vi "INVENTORY.vi"(9 "CURRENT_YEAR_DATA":string, 10 "ECODE 2":string, 11 "connection reference":T1) -> ()   [LabVIEW 2015]
uses:
  <vilib>/addons/database/Connection.llb/Conn ObjectReference.ctl
  <vilib>/Utility/miscctls.llb/LVRowAndColumnUnsignedTypeDef.ctl
  Controls/INVENTORY.ctl
  <vilib>/addons/database/Connection.llb/Conn Execute.vi
  <vilib>/addons/database/Recordset.llb/Rec Destroy - Connection.vi
  <vilib>/addons/database/_DB Variant To Data/Database Variant To Data.xnode
  <vilib>/addons/database/NI_Database_API.lvlib
  <vilib>/addons/database/Connection.llb/DB Tools Open Connec (String).vi
panel:
  out "COUNTER":dbl
  out "ECODE":string
  in  "QR_CODE (F2)":string
  in  "BOTTON_IMPORT":bool
  in  "BUTTON_EXIT":bool
  in  "Tab Control":enum32{"FROM CHECK STOCK", "FROM EXCEL FILE"}(tab)
  in  "Product":string(combo)
  in  "Path":path
  in  "NO.":string(combo)
  out "Table":string[][](table)
  # "INVENTORY"
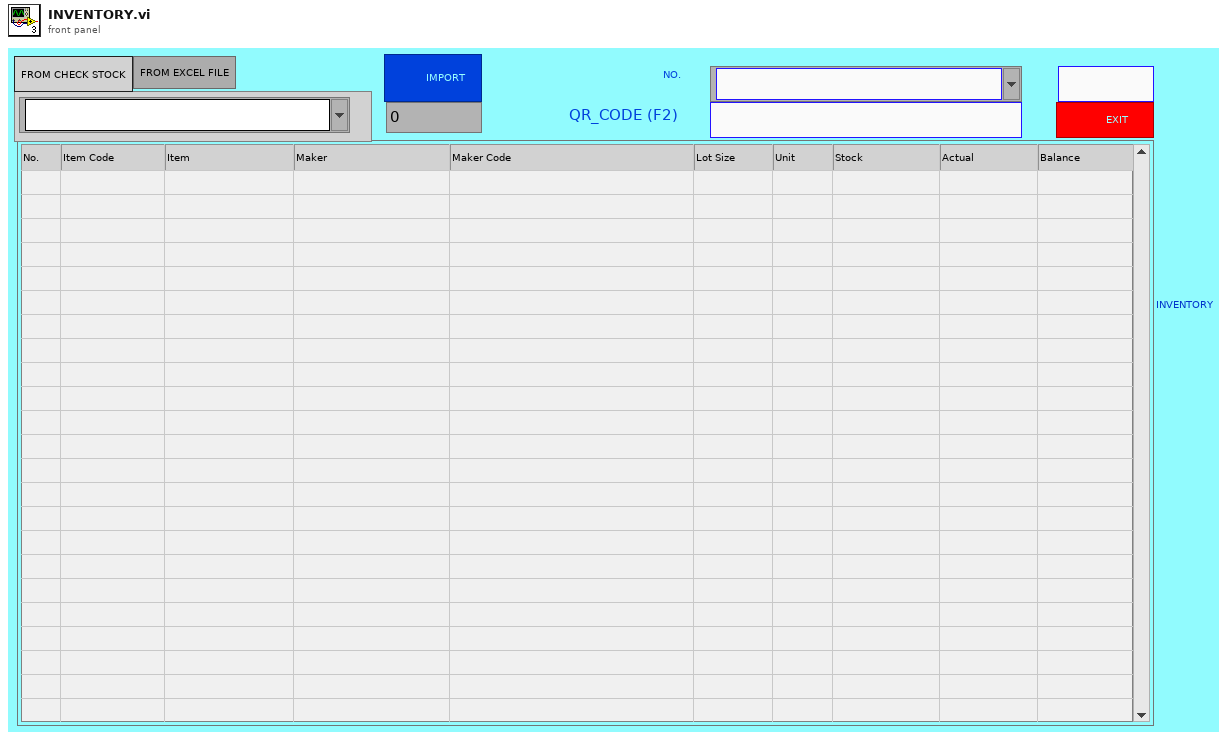
[diagram p1: front panel]
types:
  T1 = typedef "NI_Database_API.lvlib/Conn ObjectReference.ctl" = refnum<k1>
  T2 = typedef "LVRowAndColumnUnsignedTypeDef.ctl" = cluster{"Row":u32, "Column":u32}
  T3 = typedef "INVENTORY.ctl" = cluster{"ITEM_CODE":string, "PART_NAME":string, "MAKER":string, "PART_NO":string, "LOT_SIZE":dbl, "UNIT":string, "STOCK":dbl, "ACTUAL":dbl, "BALANCE":dbl}
  T4 = cluster{"QUANTITY":dbl, "INPUT_NO":string, "LINEBACK_NO":string, "OUTPUT_NO":string}[]
  T5 = cluster{"start (-1, -1)":cluster{"row":i32, "column":i32}, "end (-1, -1)":cluster{"row":i32, "column":i32}}
  T6 = cluster{"ITEM_CODE":string, "PART_NAME":string, "MAKER":string, "PART_NO":string, "LOT_SIZE":string, "UNIT":string, "STOCK":string, "ACTUAL":string, "BALANCE":string}
  T7 = cluster{"ITEM_CODE":string, "STOCK":dbl, "ACTUAL":dbl, "BALANCE":dbl}[]
  T8 = cluster{"seconds since 1Jan1904":timestamp, "NO.":string, "ECODE":string}
  T9 = typedef "NI_Database_API.lvlib/Rec ObjectReference.ctl" = refnum<k1>
  T10 = cluster{"seconds since 1Jan1904":timestamp, "String":string, "ECODE":string}
  T11 = cluster{"ITEM_CODE":string, "STOCK":dbl, "ACTUAL":dbl, "BALANCE":dbl}
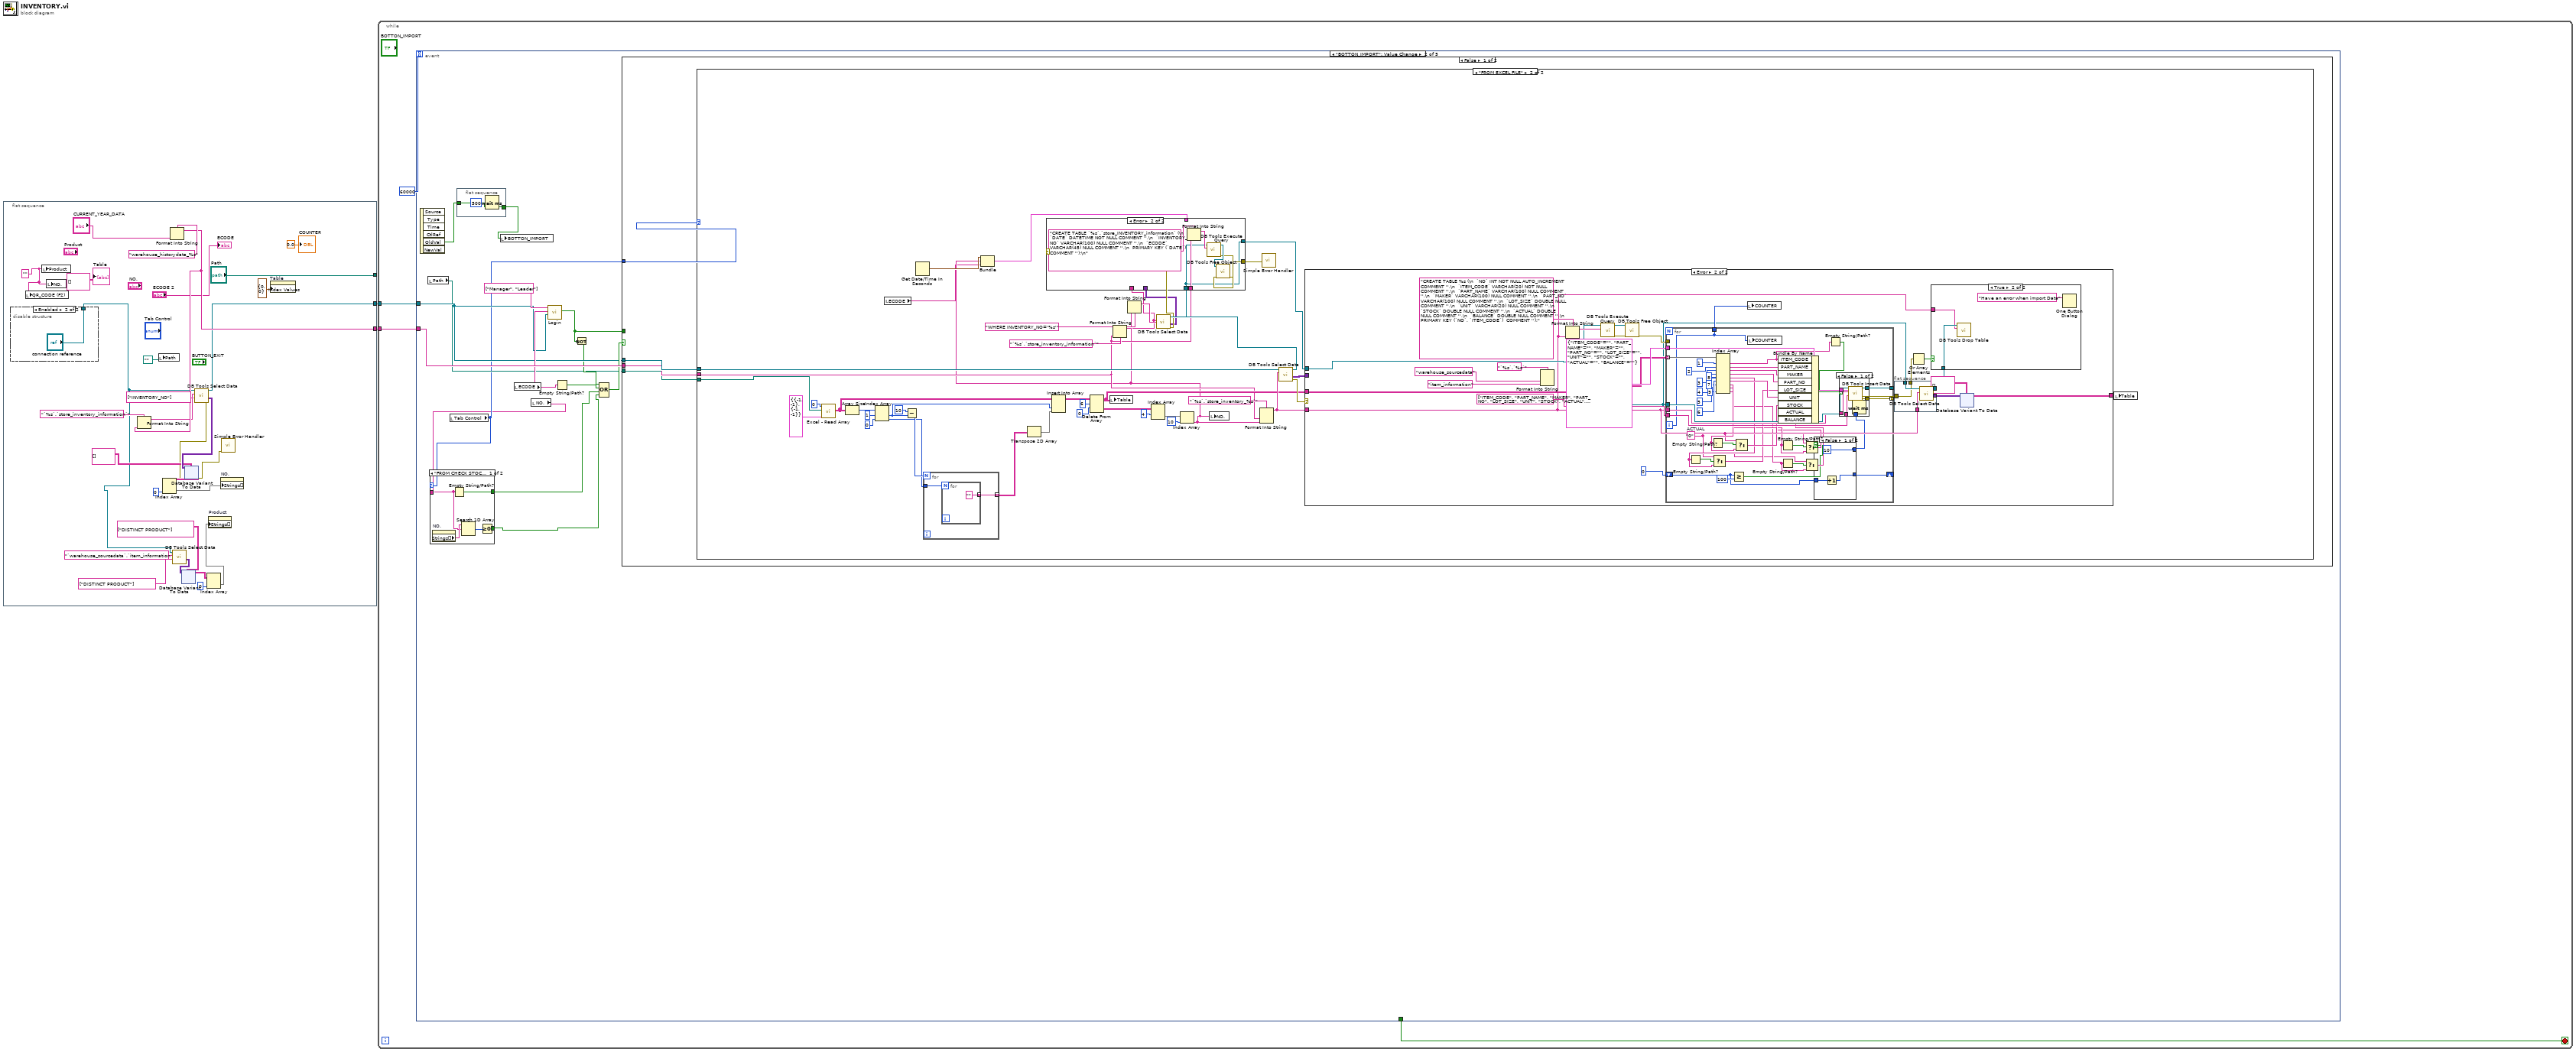
[diagram p0: block diagram]
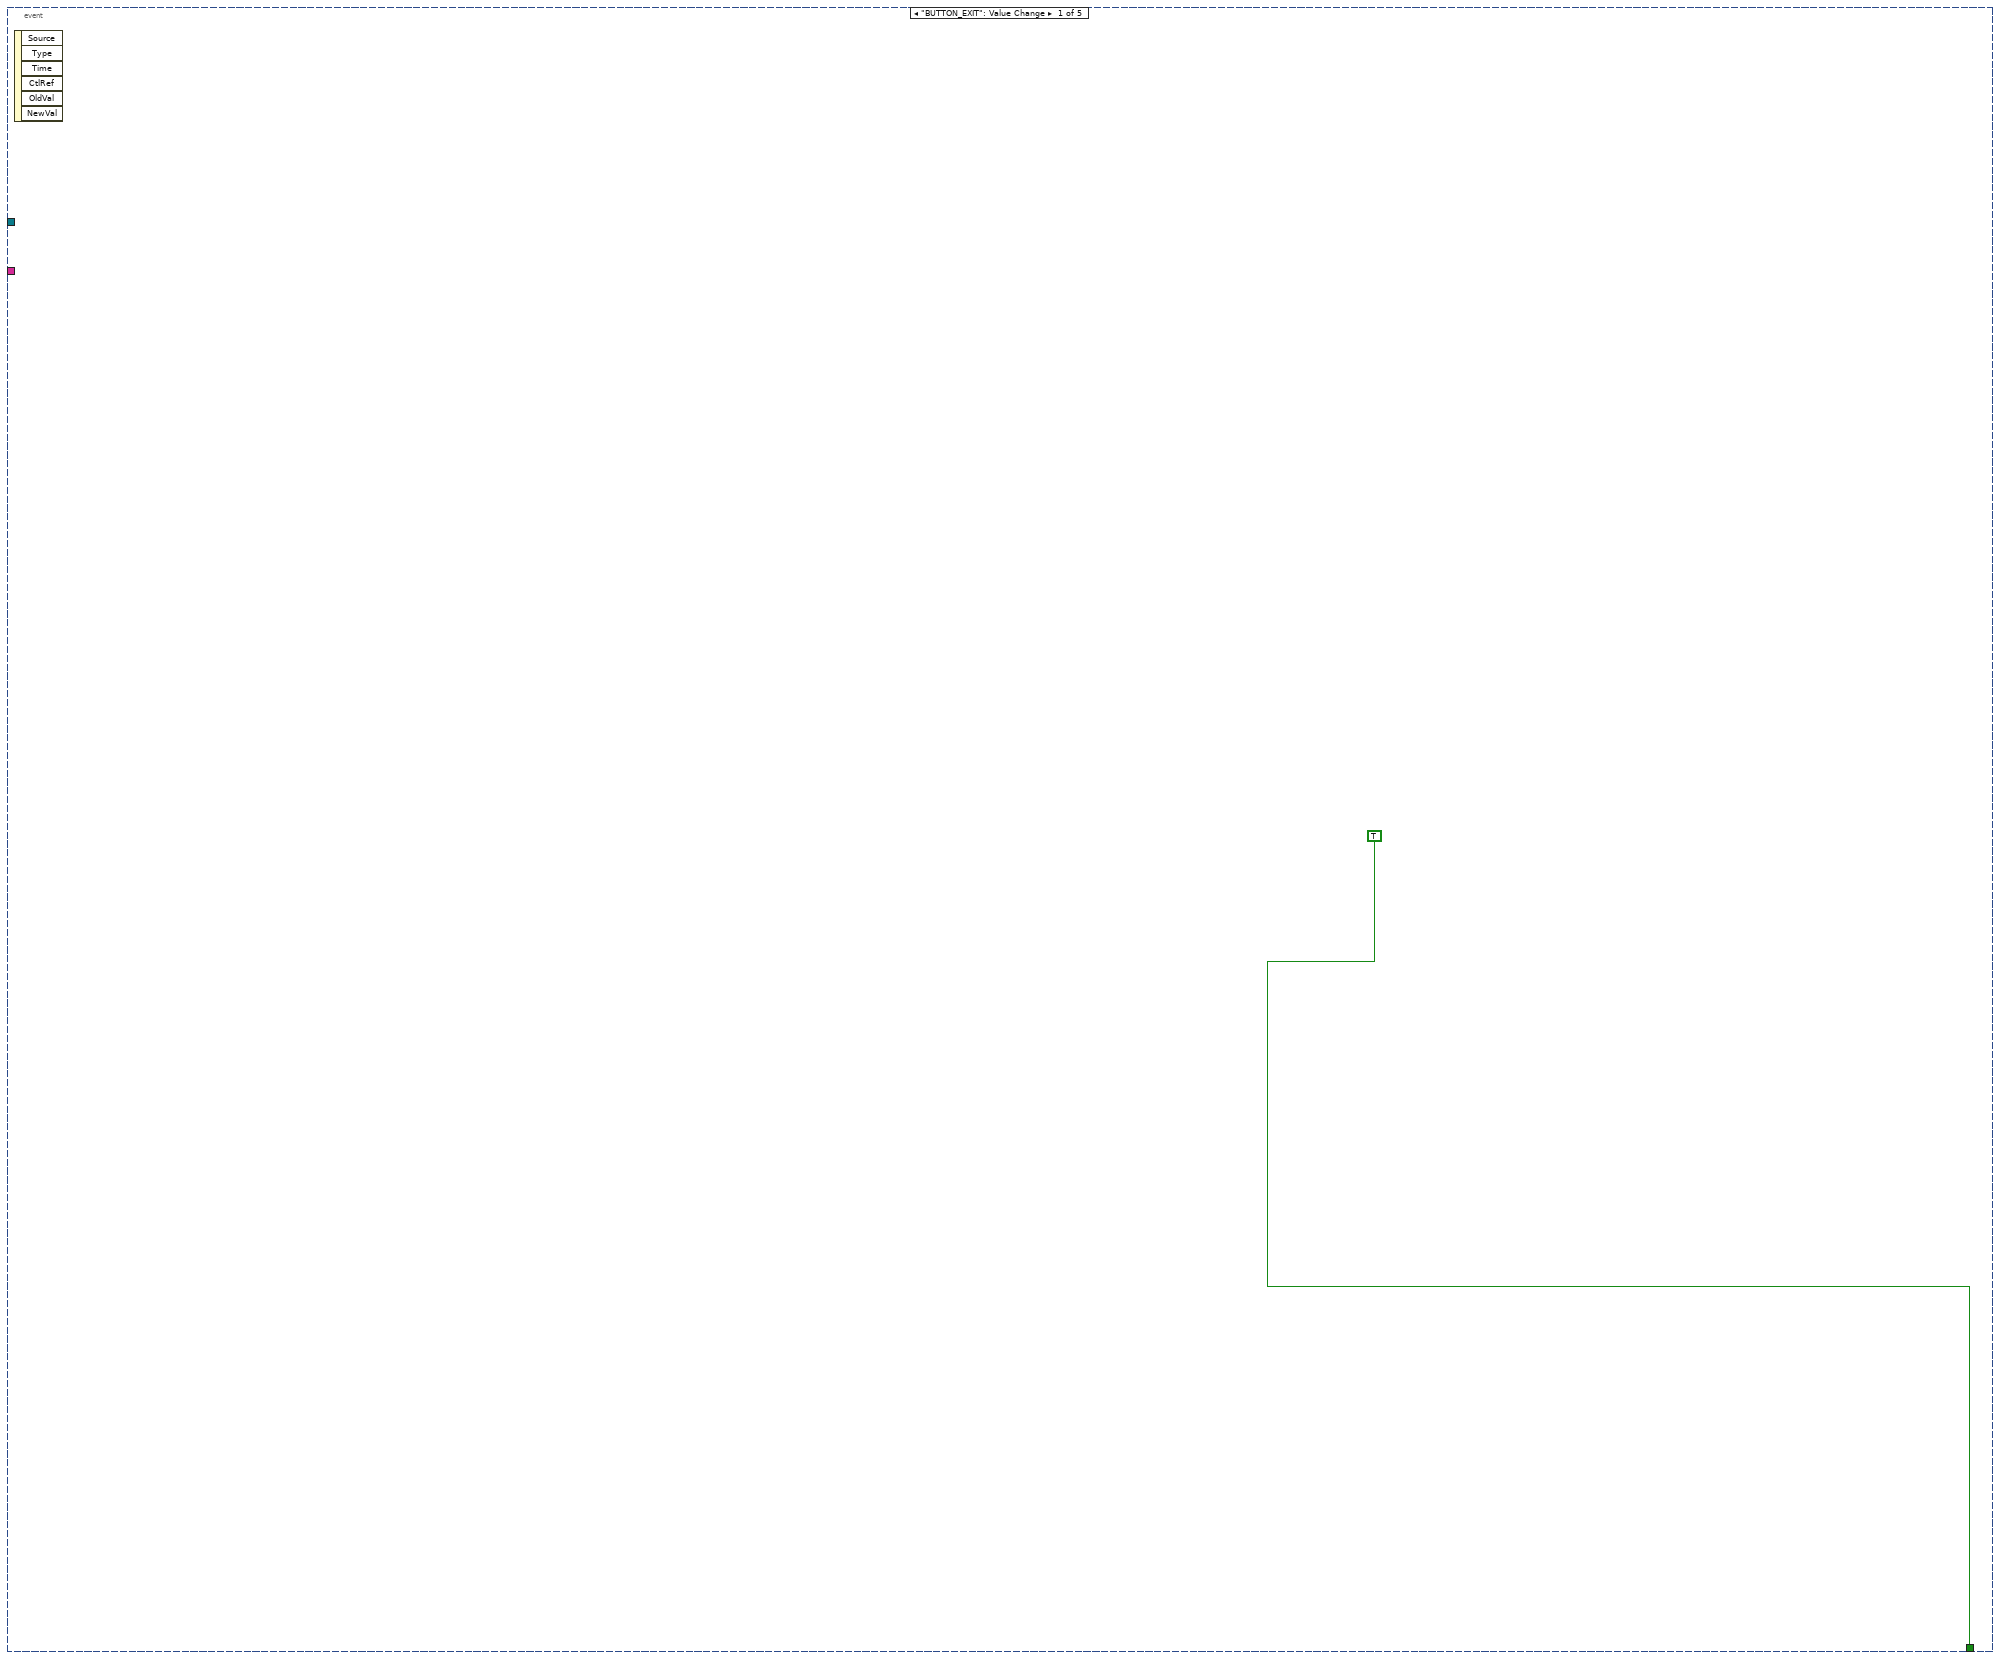
[diagram p2: hidden frame]
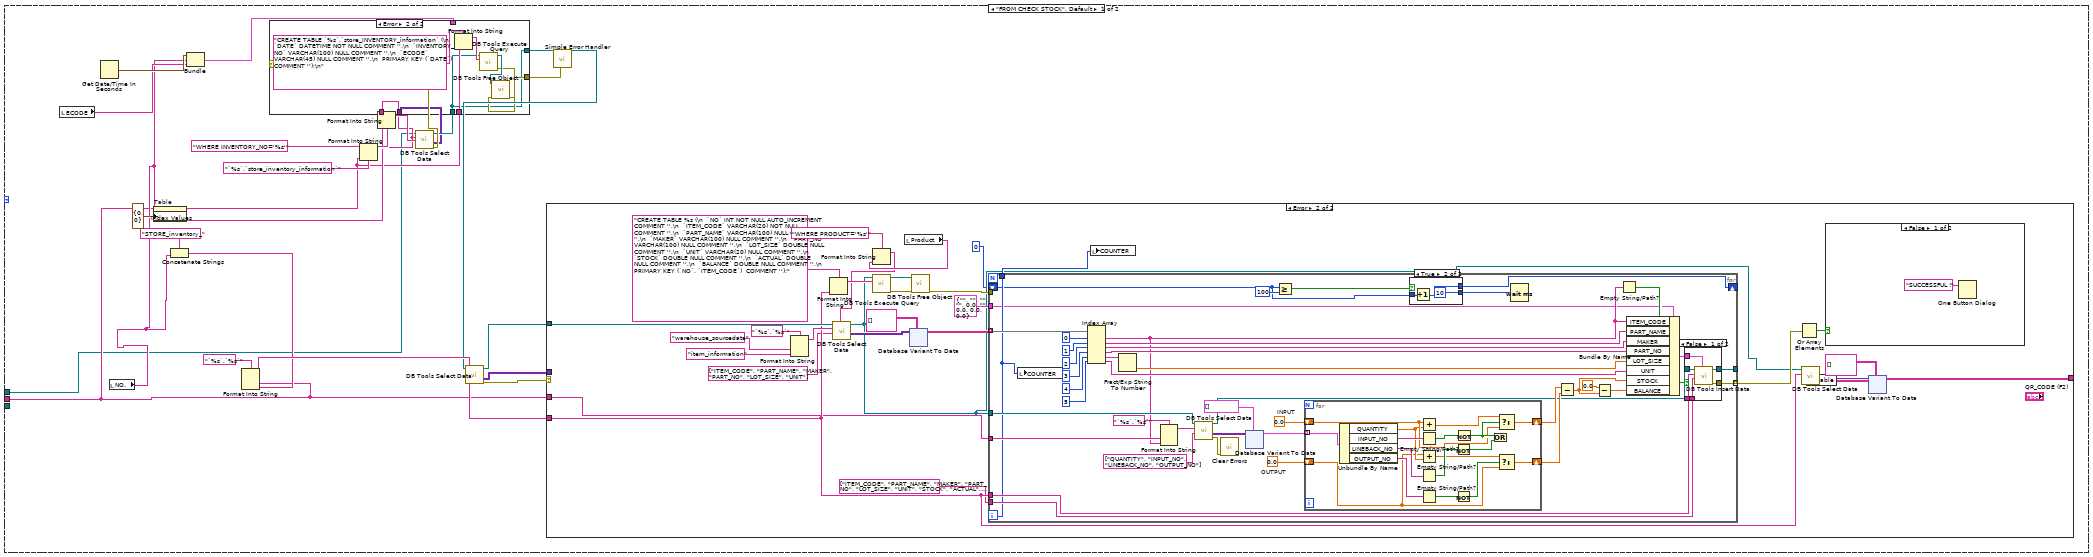
[diagram p4: hidden frame]
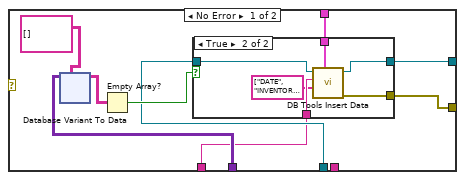
[diagram p5: hidden frame]
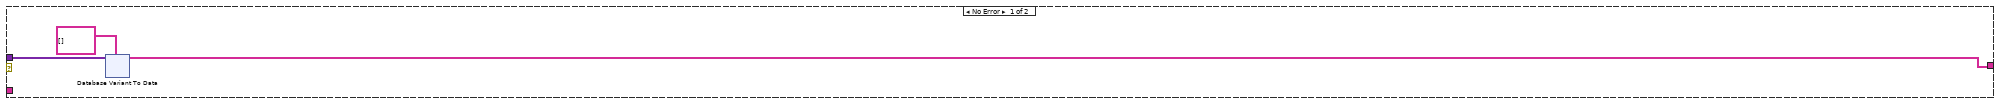
[diagram p7: hidden frame]
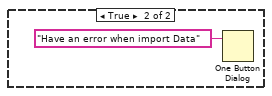
[diagram p8: hidden frame]
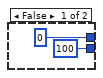
[diagram p9: hidden frame]
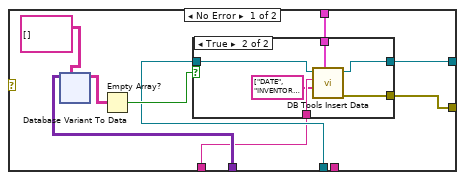
[diagram p11: hidden frame]
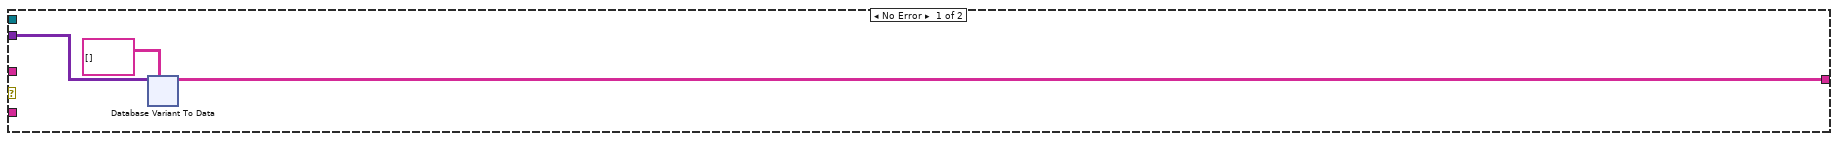
[diagram p13: hidden frame]
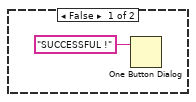
[diagram p14: hidden frame]
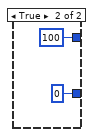
[diagram p15: hidden frame]
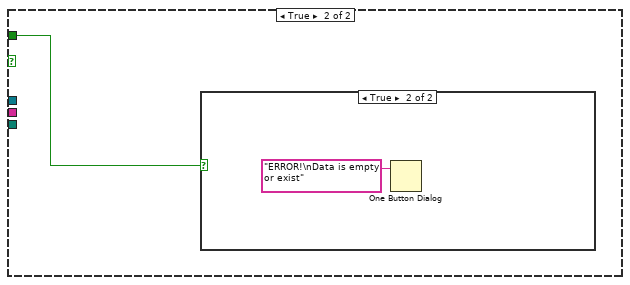
[diagram p17: hidden frame]
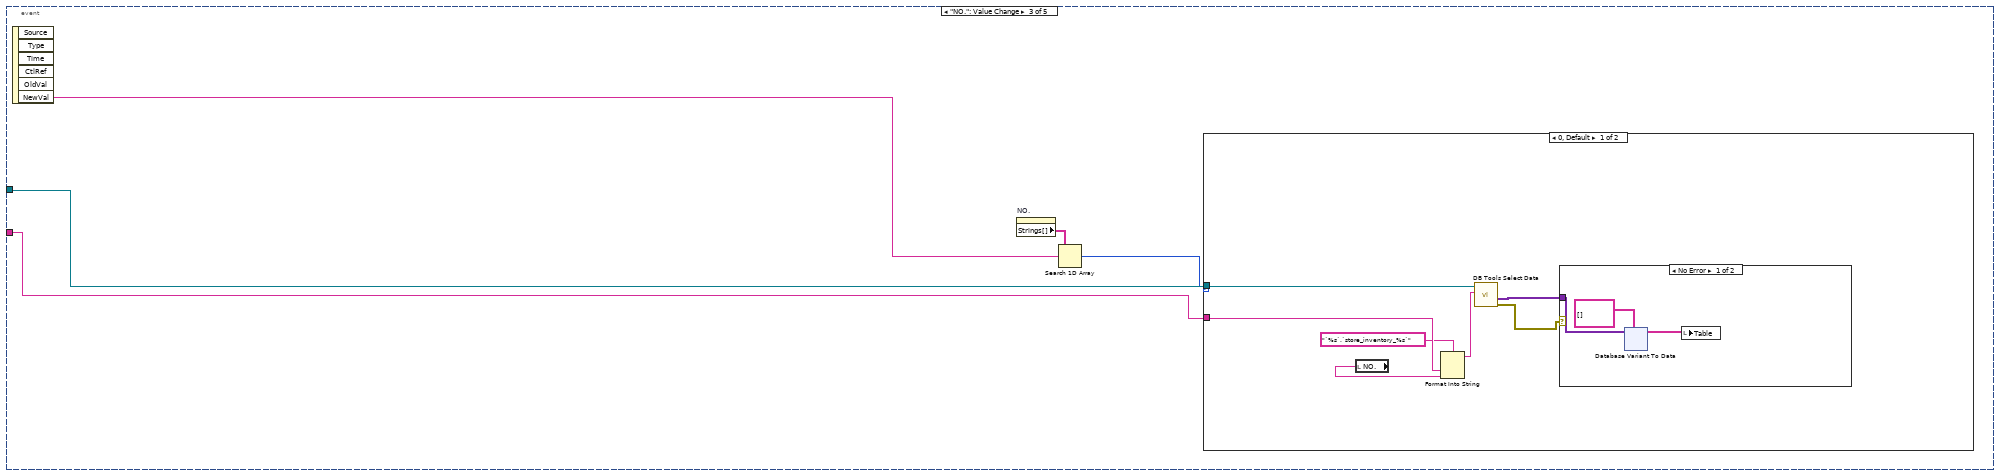
[diagram p19: hidden frame]
diagram:
  n1 = flat-sequence {
    tunnel: [w25] -> w2
    tunnel: [w28] -> w1
    tunnel: ["Path"] -> _
    frame #0 {
      w6 = ""
      n2 = disable-structure shown="Enabled" {
        disable-tunnel: [w32 "connection reference"] -> w15
        frame Disabled {
          n3 = call-poly <vilib>:"DB Tools Open Connection.vi"("password"="871994" ("userID"), "userID"="hoangbao2106", "connection information"="Database" ("userID")) -> ("connection reference"=w32:T1)  [unwired: 5 in, 1 out]
        }
        frame Enabled {
        }
      }
      n4 = local write "QR_CODE (F2)"(w6) -> ()
      n5 = local write "Product"(w6) -> ()
      n6 = local write "NO."(w6) -> ()
      n7 = local write "Path"(path "" ("Path")) -> ()
      n8 = Format Into String(format string="warehouse_historydata_%s" ("table"), "CURRENT_YEAR_DATA") -> (resulting string=w28:string)  [unwired: 2 in, 1 out]
      n9 = Format Into String(format string="`%s`.`store_inventory_information`" ("table"), w28) -> (resulting string=w27:string)  [unwired: 2 in, 1 out]
      n10 = call <vilib>:"DB Tools Select Data.vi"("columns"=string[] ["DISTINCT PRODUCT"], "table"="`warehouse_sourcedata`.`item_information`", "connection reference"=w15) -> ("data"=w14:variant[][])  [unwired: 3 in, 2 out]
      n11 = xnode "Database Variant To Data"("database variant"=w14, "type"=string[][] [["DISTINCT PRODUCT"]] ("columns")) -> ("data"=w12:string[][])  [unwired: 1 in, 1 out]
      n12 = call <vilib>:"DB Tools Select Data.vi"("columns"=string[] ["INVENTORY_NO"], "table"=w27, "connection reference"=w15) -> ("error out"=w19:errorcluster, "data"=w24:variant[][], "connection reference out"=w25:T1)  [unwired: 3 in]
      n13 = xnode "Database Variant To Data"("database variant"=w24, "error in (no error)"=w19, "type"=string[][] []) -> ("data"=w22:string[][], "error out"=w18:errorcluster)
      n14 = Index Array(array=w22, index (col)=0 ("disabled index (col)")) -> (element=w20:string[])  [unwired: 1 in]
      n15 = Index Array(array=w12, index (col)=0 ("disabled index (col)")) -> (element=w10:string[])  [unwired: 1 in]
      n16 = property on="Product" class="CmbBox"("Strings[]"=w10) -> ()  [unwired: 2 in, 2 out]
      n17 = property on="NO." class="CmbBox"("Strings[]"=w20) -> ()  [unwired: 2 in, 2 out]
      n18 = call <vilib>:"Simple Error Handler.vi"("error in (no error)"=w18) -> ()  [unwired: 4 in, 5 out]
      n19 = property on="Table" class="Tbl (strict)"("Index Values"=T2 {"Row"=0, "Column"=0}) -> ()  [unwired: 2 in, 2 out]
      "Table" <- string[][] [] ("Table")
      "ECODE" <- "ECODE 2"
      "COUNTER" <- 0.0 ("COUNTER")
    }
  }
  n20 = while {
    tunnel: w2 -> [w127]
    tunnel: w1 -> [w126]
    stop <- w128 stop-if-true
    n21 = event shown="[1] \"BOTTON_IMPORT\": Value Change" {
      selector: _ -> [_ _ _ _ _]
      dyn-events: _ -> [_ _ _ _ _]
      timeout: 60000 -> [_ _ _ _ _]
      tunnel: [TRUE _ _ _ _] -> w128
      tunnel: w127 -> [_ w139 w914 w988 w1207]
      tunnel: w126 -> [_ w144 w915 w989 w1206]
      event "BUTTON_EXIT": Value Change {
        n22 = event-data() -> ()  [unwired: 1 in, 6 out]
      }
      event "BOTTON_IMPORT": Value Change {
        n23 = event-data() -> ("OldVal"=w134:bool)  [unwired: 1 in, 5 out]
        n24 = local read "Path"() -> (w136:path)
        n25 = local read "Tab Control"() -> (w133:enum32{"FROM CHECK STOCK", "FROM EXCEL FILE"})
        n26 = flat-sequence {
          tunnel: [w151] -> w135
          tunnel: w134 -> [w151]
          frame #0 {
            n27 = Wait (ms)(milliseconds to wait=u32 500) -> ()  [unwired: 1 out]
          }
        }
        n28 = local write "BOTTON_IMPORT"(w135) -> ()
        n29 = local read "ECODE"() -> (w140:string)
        n30 = local read "NO."() -> (w132:string)
        n31 = case shown="\"FROM CHECK STOCK\", Default" w133 {
          tunnel: w132 -> [w146 _]
          tunnel: [w149 _] -> w131
          tunnel: [w145 _] -> w130
          frame "FROM CHECK STOCK", Default {
            n32 = property on="NO." class="CmbBox"() -> ("Strings[]"=w147:string[])  [unwired: 2 in, 2 out]
            n33 = Empty String/Path?(string/path=w146) -> (empty?=w149:bool)
            n34 = Search 1D Array(1D array=w147, element=w146) -> (index of element=w148:i32)  [unwired: 1 in]
            n35 = Greater Or Equal To 0?(x=w148) -> (x >= 0?=w145:bool)
          }
          frame "FROM EXCEL FILE" {
          }
        }
        n36 = call "Login.vi"("connection reference"=w139, "ACCOUNT:"=w140, "Permission"=string[] ["Manager", "Leader"]) -> ("OK"=w137:bool)  [unwired: 7 in, 1 out]
        n37 = Empty String/Path?(string/path=w140) -> (empty?=w143:bool)
        n38 = Not(x=w137) -> (.not. x?=w138:bool)
        n39 = Compound Arithmetic op=OR(w138, w143, w131, w130) -> (w142:bool)
        n40 = case shown="False" w142 {
          tunnel: w139 -> [w155 _]
          tunnel: w144 -> [w154 _]
          tunnel: w136 -> [w153 _]
          tunnel: w137 -> [_ w909]
          tunnel: w133 -> [w152 _]
          frame False {
            n41 = case shown="\"FROM EXCEL FILE\"" w152 {
              tunnel: w155 -> [w158 w640]
              tunnel: w154 -> [w159 w630]
              tunnel: w153 -> [_ w645]
              frame "FROM CHECK STOCK", Default {
                n42 = local read "ECODE"() -> (w163:string)
                n43 = Get Date/Time In Seconds() -> (seconds since 1Jan1904=w164:timestamp)
                n44 = local read "NO."() -> (w160:string)
                n45 = property on="Table" class="Tbl (strict)"("Index Values"=T2 {"Row"=0, "Column"=0}) -> ()  [unwired: 2 in, 2 out]
                n46 = Concatenate Strings("STORE_inventory_" ("string"), w160) -> (w171:string)
                n47 = Bundle("seconds since 1Jan1904"=w164, "NO."=w160, "ECODE"=w163) -> (w156:T8)  [unwired: 1 in]
                n48 = Format Into String(format string="`%s`.`%s`" ("table"), w159, w171) -> (resulting string=w174:string)  [unwired: 2 in, 1 out]
                n49 = Format Into String(format string="`%s`.`store_inventory_information`" ("table"), w159) -> (resulting string=w162:string)  [unwired: 2 in, 1 out]
                n50 = Format Into String(format string="WHERE INVENTORY_NO='%s'" ("table"), w160) -> (resulting string=w166:string)  [unwired: 2 in, 1 out]
                n51 = call <vilib>:"DB Tools Select Data.vi"("condition"=w166, "table"=w162, "connection reference"=w158) -> ("error out"=w169:errorcluster, "data"=w165:variant[][], "connection reference out"=w168:T1)  [unwired: 3 in]
                n52 = case shown="Error" w169 {
                  tunnel: w168 -> [w184 w240]
                  tunnel: w159 -> [_ w245]
                  tunnel: [w181 w241] -> w161
                  tunnel: w165 -> [w188 _]
                  tunnel: w156 -> [w183 _]
                  tunnel: w162 -> [w182 _]
                  tunnel: [w180 w240] -> w157
                  frame No Error {
                    n53 = xnode "Database Variant To Data"("database variant"=w188, "type"=string[][] []) -> ("data"=w186:string[][])  [unwired: 1 in, 1 out]
                    n54 = Empty Array?(array=w186) -> (empty?=w185:bool)
                    n55 = case shown="True" w185 {
                      tunnel: w184 -> [w189 w195]
                      tunnel: w183 -> [_ w194]
                      tunnel: w182 -> [_ w193]
                      tunnel: [_ w191] -> w181
                      tunnel: [w189 w190] -> w180
                      frame False {
                      }
                      frame True {
                        n56 = call <vilib>:"DB Tools Insert Data.vi"("data"=w194, "columns"=string[] ["DATE", "INVENTORY_NO", "ECODE"], "table"=w193, "connection reference"=w195) -> ("error out"=w191:errorcluster, "connection reference out"=w190:T1)  [unwired: 6 in]
                      }
                    }
                  }
                  frame Error {
                    n57 = Format Into String(format string="CREATE TABLE `%s`.`store_INVENTORY_information` (\n  `DATE` DATETIME NOT NULL COMMENT '',\n  `INVENTORY_NO` VARCHAR(100) NULL COMMENT '',\n  `ECODE` VARCHAR(45) NULL COMMENT '',\n  PRIMARY KEY (`DATE`)  COMMENT '');\n" ("SQL query"), w245) -> (resulting string=w244:string)  [unwired: 2 in, 1 out]
                    n58 = call-poly <vilib>:"DB Tools Execute Query.vi"("SQL query"=w244, "connection reference"=w240) -> ("error out"=w242:errorcluster, "recordset reference"=w243:T9)  [unwired: 6 in]
                    n59 = call-poly <vilib>:"DB Tools Free Object.vi"("error in (no error)"=w242, "recordset reference"=w243) -> ("error out"=w241:errorcluster)  [unwired: 8 in, 1 out]
                  }
                }
                n60 = call <vilib>:"DB Tools Select Data.vi"("table"=w174, "connection reference"=w157) -> ("error out"=w178:errorcluster, "data"=w177:variant[][], "connection reference out"=w176:T1)  [unwired: 4 in]
                n61 = case shown="Error" w178 {
                  tunnel: w177 -> [w247 _]
                  tunnel: w176 -> [_ w318]
                  tunnel: w174 -> [_ w307]
                  tunnel: [w248 w306] -> w175
                  tunnel: w159 -> [_ w303]
                  frame No Error {
                    n62 = xnode "Database Variant To Data"("database variant"=w247, "type"=string[][] []) -> ("data"=w248:string[][])  [unwired: 1 in, 1 out]
                  }
                  frame Error {
                    n63 = Format Into String(format string="`%s`.`%s`" ("table"), "warehouse_sourcedata" ("table"), "item_information" ("table")) -> (resulting string=w319:string)  [unwired: 2 in, 1 out]
                    n64 = Format Into String(format string="CREATE TABLE %s (\n  `NO` INT NOT NULL AUTO_INCREMENT COMMENT '',\n  `ITEM_CODE` VARCHAR(20) NOT NULL COMMENT '',\n  `PART_NAME` VARCHAR(100) NULL COMMENT '',\n  `MAKER` VARCHAR(100) NULL COMMENT '',\n  `PART_NO` VARCHAR(100) NULL COMMENT '',\n  `LOT_SIZE` DOUBLE NULL COMMENT '',\n  `UNIT` VARCHAR(20) NULL COMMENT '',\n  `STOCK` DOUBLE NULL COMMENT '',\n  `ACTUAL` DOUBLE NULL COMMENT '',\n  `BALANCE` DOUBLE NULL COMMENT '',\n  PRIMARY KEY (`NO`, `ITEM_CODE`)  COMMENT '');", w307) -> (resulting string=w316:string)  [unwired: 2 in, 1 out]
                    n65 = local read "Product"() -> (w296:string)
                    n66 = Format Into String(format string="WHERE PRODUCT='%s'", w296) -> (resulting string=w295:string)  [unwired: 2 in, 1 out]
                    n67 = call <vilib>:"DB Tools Select Data.vi"("condition"=w295, "columns"=string[] ["ITEM_CODE", "PART_NAME", "MAKER", "PART_NO", "LOT_SIZE", "UNIT"], "table"=w319, "connection reference"=w318) -> ("data"=w315:variant[][], "connection reference out"=w298:T1)  [unwired: 2 in, 1 out]
                    n68 = call-poly <vilib>:"DB Tools Execute Query.vi"("SQL query"=w316, "connection reference"=w298) -> ("error out"=w309:errorcluster, "recordset reference"=w311:T9)  [unwired: 6 in]
                    n69 = xnode "Database Variant To Data"("database variant"=w315, "type"=string[][] []) -> ("data"=w304:string[][])  [unwired: 1 in, 1 out]
                    n70 = call-poly <vilib>:"DB Tools Free Object.vi"("error in (no error)"=w309, "recordset reference"=w311) -> ("error out"=w310:errorcluster)  [unwired: 8 in, 1 out]
                    n71 = for {
                      tunnel: w298 -> [w440]
                      tunnel: string[] ["ITEM_CODE", "PART_NAME", "MAKER", "PART_NO", "LOT_SIZE", "UNIT", "STOCK", "ACTUAL", "BALANCE"] ("columns") -> [w456]
                      tunnel: [w455] -> w313 mode=indexing
                      tunnel: w310 -> [_]
                      tunnel: w307 -> [w454]
                      tunnel: [w453] -> _
                      tunnel: w304 -> [w452] mode=indexing
                      tunnel: T3 {"ITEM_CODE"="", "PART_NAME"="", "MAKER"="", "PART_NO"="", "LOT_SIZE"=0.0, "UNIT"="", "STOCK"=0.0, "ACTUAL"=0.0, "BALANCE"=0.0} -> [w413]
                      tunnel: w303 -> [w438]
                      tunnel: [w421] -> w299
                      shift-right: [w414] -> _
                      shift-left: 0 -> [w415]
                      i -> [w421]
                      w431 = 0.0  # OUTPUT
                      w432 = 0.0  # INPUT
                      n72 = local write "COUNTER"(w421) -> ()
                      n73 = Index Array(array=w452, index #1=0 ("index"), index #2=1 ("index"), index #3=2 ("index"), index #4=3 ("index"), index #5=4 ("index"), index #6=5 ("index")) -> (element #1=w419:string, element #2=w445:string, element #3=w444:string, element #4=w443:string, element #5=w427:string, element #6=w442:string)
                      n74 = Fract/Exp String To Number(string=w427) -> (number=w426:dbl)  [unwired: 3 in, 1 out]
                      n75 = Format Into String(format string="`%s`.`%s`", w438, w419) -> (resulting string=w437:string)  [unwired: 2 in, 1 out]
                      n76 = call <vilib>:"DB Tools Select Data.vi"("columns"=string[] ["QUANTITY", "INPUT_NO", "LINEBACK_NO", "OUTPUT_NO"], "table"=w437, "connection reference"=w440) -> ("error out"=w422:errorcluster, "data"=w435:variant[][], "connection reference out"=w428:T1)  [unwired: 3 in]
                      n77 = call <vilib>:"Clear Errors.vi"("error in (no error)"=w422) -> ()  [unwired: 5 in, 2 out]
                      n78 = xnode "Database Variant To Data"("database variant"=w435, "type"=T4 []) -> ("data"=w433:T4)  [unwired: 1 in, 1 out]
                      n79 = Greater Or Equal?(x=w415, y=100) -> (x >= y?=w416:bool)
                      n80 = for {
                        tunnel: w433 -> [w485] mode=indexing
                        shift-right: [w477] -> w430
                        shift-left: w432 -> [w476]
                        shift-right: [w469] -> w429
                        shift-left: w431 -> [w470]
                        n81 = Unbundle By Name(w485) -> ("QUANTITY"=w472:dbl, "INPUT_NO"=w484:string, "LINEBACK_NO"=w481:string, "OUTPUT_NO"=w474:string)
                        n82 = Add(x=w476, y=w472) -> (x+y=w478:dbl)
                        n83 = Empty String/Path?(string/path=w484) -> (empty?=w483:bool)
                        n84 = Add(x=w470, y=w472) -> (x+y=w471:dbl)
                        n85 = Empty String/Path?(string/path=w481) -> (empty?=w482:bool)
                        n86 = Empty String/Path?(string/path=w474) -> (empty?=w475:bool)
                        n87 = Not(x=w482) -> (.not. x?=w480:bool)
                        n88 = Not(x=w475) -> (.not. x?=w473:bool)
                        n89 = Not(x=w483) -> (.not. x?=w479:bool)
                        n90 = Or(x=w479, y=w480) -> ()  [unwired: 1 out]
                        n91 = Select(t=w478, s=w479, f=w476) -> (s? t:f=w477:dbl)
                        n92 = Select(t=w471, s=w473, f=w470) -> (s? t:f=w469:dbl)
                      }
                      n93 = case shown="True" w416 {
                        tunnel: [u32 100 ("milliseconds to wait") u32 10 ("milliseconds to wait")] -> w420
                        tunnel: w415 -> [_ w460]
                        tunnel: [0 w459] -> w414
                        frame False {
                        }
                        frame True {
                          n94 = Increment(x=w460) -> (x+1=w459:i32)
                        }
                      }
                      n95 = Wait (ms)(milliseconds to wait=w420) -> ()  [unwired: 1 out]
                      n96 = Subtract(x=w430, y=w429) -> (x-y=w424:dbl)
                      n97 = Subtract(x=0.0, y=w424) -> (x-y=w423:dbl)
                      n98 = Empty String/Path?(string/path=w419) -> (empty?=w418:bool)
                      n99 = Bundle By Name(cluster=w413, "ITEM_CODE"=w419, "PART_NAME"=w445, "MAKER"=w444, "PART_NO"=w443, "LOT_SIZE"=w426, "UNIT"=w442, "STOCK"=w424, "BALANCE"=w423) -> (w441:T3)
                      n100 = case shown="False" w418 {
                        tunnel: w456 -> [w467 _]
                        tunnel: [w466 _] -> w455
                        tunnel: w454 -> [w465 _]
                        tunnel: [w464 w468] -> w453
                        tunnel: w441 -> [w463 _]
                        tunnel: w428 -> [w462 w468]
                        frame False {
                          n101 = call <vilib>:"DB Tools Insert Data.vi"("data"=w463, "columns"=w467, "table"=w465, "connection reference"=w462) -> ("error out"=w466:errorcluster, "connection reference out"=w464:T1)  [unwired: 6 in]
                        }
                        frame True {
                        }
                      }
                    }
                    n102 = local write "COUNTER"(w299) -> ()
                    n103 = Or Array Elements(Boolean array=w313) -> (logical OR=w312:bool)
                    n104 = call <vilib>:"DB Tools Select Data.vi"("table"=w307, "connection reference"=w298) -> ("data"=w301:variant[][])  [unwired: 4 in, 2 out]
                    n105 = case shown="False" w312 {
                      frame False {
                        n106 = One Button Dialog(message="SUCCESSFUL !") -> ()  [unwired: 1 in, 1 out]
                      }
                      frame True {
                        n107 = One Button Dialog(message="Have an error when import Data") -> ()  [unwired: 1 in, 1 out]
                      }
                    }
                    n108 = xnode "Database Variant To Data"("database variant"=w301, "type"=string[][] []) -> ("data"=w306:string[][])  [unwired: 1 in, 1 out]
                  }
                }
                n109 = call <vilib>:"Simple Error Handler.vi"("error in (no error)"=w161) -> ()  [unwired: 4 in, 5 out]
                n110 = local write "Table"(w175) -> ()
              }
              frame "FROM EXCEL FILE" {
                n111 = call "Excel - Read Array.vi"("Cluster"=T5 {"start (-1, -1)"={"row"=-1, "column"=-1}, "end (-1, -1)"={"row"=-1, "column"=-1}}, "Path"=w645, "worksheet index (0)"=0) -> ("Element 1"=w642:string[][])  [unwired: 5 in, 1 out]
                n112 = Array Size(array=w642) -> (size(s)=w655:i32[])
                n113 = Index Array(array=w655, index #1=1 ("index"), index #2=0 ("index")) -> (element #1=w647:i32, element #2=w650:i32)
                n114 = local read "ECODE"() -> (w624:string)
                n115 = Subtract(x=10, y=w647) -> (x-y=w653:i32)
                n116 = Get Date/Time In Seconds() -> (seconds since 1Jan1904=w626:timestamp)
                n117 = for {
                  N: w653 -> [_]
                  tunnel: [w907] -> w649 mode=indexing
                  tunnel: w650 -> [w906]
                  n118 = for {
                    N: w906 -> [_]
                    tunnel: [""] -> w907 mode=indexing
                  }
                }
                n119 = Transpose 2D Array(2D array=w649) -> (transposed array=w648:string[][])
                n120 = Insert Into Array(array=w642, index (col)=w647, new element=w648) -> (w646:string[][])  [unwired: 1 in]
                n121 = Delete From Array(array=w646, length=6, index (row)=0 ("disabled index (col)")) -> (deleted portion=w656:string[][], array with subset deleted=w635:string[][])  [unwired: 1 in]
                n122 = local write "Table"(w635) -> ()
                n123 = Format Into String(format string="`%s`.`store_inventory_information`" ("table"), w630) -> (resulting string=w622:string)  [unwired: 2 in, 1 out]
                n124 = Index Array(array=w656, index (row)=4) -> (element=w660:string[])  [unwired: 1 in]
                n125 = Index Array(array=w660, index=10) -> (element=w625:string)
                n126 = Bundle("seconds since 1Jan1904"=w626, "String"=w625, "ECODE"=w624) -> (w623:T10)  [unwired: 1 in]
                n127 = Format Into String(format string="WHERE INVENTORY_NO='%s'" ("table"), w625) -> (resulting string=w628:string)  [unwired: 2 in, 1 out]
                n128 = local write "NO."(w625) -> ()
                n129 = Format Into String(format string="`%s`.`store_inventory_%s`" ("table"), w630, w625) -> (resulting string=w638:string)  [unwired: 2 in, 1 out]
                n130 = call <vilib>:"DB Tools Select Data.vi"("table"=w638, "connection reference"=w640) -> ("error out"=w639:errorcluster, "data"=w636:variant[][], "connection reference out"=w634:T1)  [unwired: 4 in]
                n131 = call <vilib>:"DB Tools Select Data.vi"("condition"=w628, "table"=w622, "connection reference"=w634) -> ("error out"=w632:errorcluster, "data"=w627:variant[][], "connection reference out"=w631:T1)  [unwired: 3 in]
                n132 = case shown="Error" w632 {
                  tunnel: w631 -> [w666 w722]
                  tunnel: w630 -> [_ w727]
                  tunnel: [w663 w723] -> w621
                  tunnel: w627 -> [w670 _]
                  tunnel: w623 -> [w665 _]
                  tunnel: w622 -> [w664 _]
                  tunnel: [w662 w722] -> w620
                  frame No Error {
                    n133 = xnode "Database Variant To Data"("database variant"=w670, "type"=string[][] []) -> ("data"=w668:string[][])  [unwired: 1 in, 1 out]
                    n134 = Empty Array?(array=w668) -> (empty?=w667:bool)
                    n135 = case shown="True" w667 {
                      tunnel: w666 -> [w671 w677]
                      tunnel: w665 -> [_ w676]
                      tunnel: w664 -> [_ w675]
                      tunnel: [_ w673] -> w663
                      tunnel: [w671 w672] -> w662
                      frame False {
                      }
                      frame True {
                        n136 = call <vilib>:"DB Tools Insert Data.vi"("data"=w676, "columns"=string[] ["DATE", "INVENTORY_NO", "ECODE"], "table"=w675, "connection reference"=w677) -> ("error out"=w673:errorcluster, "connection reference out"=w672:T1)  [unwired: 6 in]
                      }
                    }
                  }
                  frame Error {
                    n137 = Format Into String(format string="CREATE TABLE `%s`.`store_INVENTORY_information` (\n  `DATE` DATETIME NOT NULL COMMENT '',\n  `INVENTORY_NO` VARCHAR(100) NULL COMMENT '',\n  `ECODE` VARCHAR(45) NULL COMMENT '',\n  PRIMARY KEY (`DATE`)  COMMENT '');\n" ("SQL query"), w727) -> (resulting string=w726:string)  [unwired: 2 in, 1 out]
                    n138 = call-poly <vilib>:"DB Tools Execute Query.vi"("SQL query"=w726, "connection reference"=w722) -> ("error out"=w724:errorcluster, "recordset reference"=w725:T9)  [unwired: 6 in]
                    n139 = call-poly <vilib>:"DB Tools Free Object.vi"("error in (no error)"=w724, "recordset reference"=w725) -> ("error out"=w723:errorcluster)  [unwired: 8 in, 1 out]
                  }
                }
                n140 = call <vilib>:"Simple Error Handler.vi"("error in (no error)"=w621) -> ()  [unwired: 4 in, 5 out]
                n141 = case shown="Error" w639 {
                  tunnel: w636 -> [w730 _]
                  tunnel: w620 -> [_ w781]
                  tunnel: w638 -> [_ w777]
                  tunnel: [w729 w786] -> w637
                  tunnel: w635 -> [_ w783]
                  frame No Error {
                    n142 = xnode "Database Variant To Data"("database variant"=w730, "type"=string[][] []) -> ("data"=w729:string[][])  [unwired: 1 in, 1 out]
                  }
                  frame Error {
                    n143 = Format Into String(format string="`%s`.`%s`" ("table"), "warehouse_sourcedata" ("table"), "item_information" ("table")) -> ()  [unwired: 2 in, 2 out]
                    n144 = Format Into String(format string="CREATE TABLE %s (\n  `NO` INT NOT NULL AUTO_INCREMENT COMMENT '',\n  `ITEM_CODE` VARCHAR(20) NOT NULL COMMENT '',\n  `PART_NAME` VARCHAR(100) NULL COMMENT '',\n  `MAKER` VARCHAR(100) NULL COMMENT '',\n  `PART_NO` VARCHAR(100) NULL COMMENT '',\n  `LOT_SIZE` DOUBLE NULL COMMENT '',\n  `UNIT` VARCHAR(20) NULL COMMENT '',\n  `STOCK` DOUBLE NULL COMMENT '',\n  `ACTUAL` DOUBLE NULL COMMENT '',\n  `BALANCE` DOUBLE NULL COMMENT '',\n  PRIMARY KEY (`NO`, `ITEM_CODE`)  COMMENT '');", w777) -> (resulting string=w793:string)  [unwired: 2 in, 1 out]
                    n145 = call-poly <vilib>:"DB Tools Execute Query.vi"("SQL query"=w793, "connection reference"=w781) -> ("error out"=w789:errorcluster, "recordset reference"=w791:T9)  [unwired: 6 in]
                    n146 = call-poly <vilib>:"DB Tools Free Object.vi"("error in (no error)"=w789, "recordset reference"=w791) -> ("error out"=w790:errorcluster)  [unwired: 8 in, 1 out]
                    n147 = for {
                      tunnel: w781 -> [w892]
                      tunnel: string[] ["ITEM_CODE", "PART_NAME", "MAKER", "PART_NO", "LOT_SIZE", "UNIT", "STOCK", "ACTUAL", "BALANCE"] ("columns") -> [w891]
                      tunnel: [w890] -> w780 mode=indexing
                      tunnel: w790 -> [_]
                      tunnel: w777 -> [w889]
                      tunnel: [w888] -> _
                      tunnel: w783 -> [w886] mode=indexing
                      tunnel: T6 {"ITEM_CODE"="", "PART_NAME"="", "MAKER"="", "PART_NO"="", "LOT_SIZE"="", "UNIT"="", "STOCK"="", "ACTUAL"="", "BALANCE"=""} -> [w887]
                      tunnel: [w873] -> w782
                      shift-right: [w852] -> _
                      shift-left: 0 -> [w853]
                      i -> [w873]
                      w858 = "0"  # ACTUAL
                      n148 = Index Array(array=w886, index #1=1 ("index"), index #2=2 ("index"), index #3=3 ("index"), index #4=4 ("index"), index #5=5 ("index"), index #6=6 ("index"), index #7=7 ("index"), index #8=8 ("index"), index #9=9 ("index")) -> (element #1=w857:string, element #2=w879:string, element #3=w878:string, element #4=w877:string, element #5=w866:string, element #6=w876:string, element #7=w869:string, element #8=w863:string, element #9=w860:string)
                      n149 = Empty String/Path?(string/path=w866) -> (empty?=w867:bool)
                      n150 = Empty String/Path?(string/path=w869) -> (empty?=w870:bool)
                      n151 = Select(t=w858, s=w867, f=w866) -> (s? t:f=w865:string)
                      n152 = Greater Or Equal?(x=w853, y=100) -> (x >= y?=w854:bool)
                      n153 = Select(t=w858, s=w870, f=w869) -> (s? t:f=w868:string)
                      n154 = local write "COUNTER"(w873) -> ()
                      n155 = Empty String/Path?(string/path=w863) -> (empty?=w864:bool)
                      n156 = Empty String/Path?(string/path=w860) -> (empty?=w861:bool)
                      n157 = Select(t=w858, s=w864, f=w863) -> (s? t:f=w862:string)
                      n158 = Select(t=w858, s=w861, f=w860) -> (s? t:f=w859:string)
                      n159 = Bundle By Name(cluster=w887, "ITEM_CODE"=w857, "PART_NAME"=w879, "MAKER"=w878, "PART_NO"=w877, "LOT_SIZE"=w865, "UNIT"=w876, "STOCK"=w868, "ACTUAL"=w862, "BALANCE"=w859) -> (w875:T6)
                      n160 = case shown="False" w854 {
                        tunnel: [u32 10 ("milliseconds to wait") u32 100 ("milliseconds to wait")] -> w851
                        tunnel: w853 -> [w894 _]
                        tunnel: [w893 0] -> w852
                        frame False {
                          n161 = Increment(x=w894) -> (x+1=w893:i32)
                        }
                        frame True {
                        }
                      }
                      n162 = Empty String/Path?(string/path=w857) -> (empty?=w856:bool)
                      n163 = case shown="False" w856 {
                        tunnel: w892 -> [w904 w905]
                        tunnel: w891 -> [w903 _]
                        tunnel: [w902 _] -> w890
                        tunnel: w889 -> [w901 _]
                        tunnel: [w900 w905] -> w888
                        tunnel: w875 -> [w899 _]
                        tunnel: w851 -> [w898 _]
                        frame False {
                          n164 = call <vilib>:"DB Tools Insert Data.vi"("data"=w899, "columns"=w903, "table"=w901, "connection reference"=w904) -> ("error out"=w902:errorcluster, "connection reference out"=w900:T1)  [unwired: 6 in]
                          n165 = Wait (ms)(milliseconds to wait=w898) -> ()  [unwired: 1 out]
                        }
                        frame True {
                        }
                      }
                    }
                    n166 = local write "COUNTER"(w782) -> ()
                    n167 = flat-sequence {
                      tunnel: [w802] -> w787
                      tunnel: w777 -> [w801]
                      tunnel: w781 -> [w800]
                      tunnel: [w799] -> w779
                      tunnel: w780 -> [w799]
                      tunnel: [w798] -> w778
                      frame #0 {
                        n168 = call <vilib>:"DB Tools Select Data.vi"("table"=w801, "connection reference"=w800) -> ("data"=w802:variant[][], "connection reference out"=w798:T1)  [unwired: 4 in, 1 out]
                      }
                    }
                    n169 = Or Array Elements(Boolean array=w779) -> (logical OR=w792:bool)
                    n170 = case shown="True" w792 {
                      tunnel: w778 -> [_ w849]
                      tunnel: w777 -> [_ w848]
                      frame False {
                        n171 = One Button Dialog(message="SUCCESSFUL !") -> ()  [unwired: 1 in, 1 out]
                      }
                      frame True {
                        n172 = call <vilib>:"DB Tools Drop Table.vi"("table"=w848, "connection reference"=w849) -> ()  [unwired: 6 in, 2 out]
                        n173 = One Button Dialog(message="Have an error when import Data") -> ()  [unwired: 1 in, 1 out]
                      }
                    }
                    n174 = xnode "Database Variant To Data"("database variant"=w787, "type"=string[][] []) -> ("data"=w786:string[][])  [unwired: 1 in, 1 out]
                  }
                }
                n175 = local write "Table"(w637) -> ()
              }
            }
          }
          frame True {
            n176 = case shown="True" w909 {
              frame False {
              }
              frame True {
                n177 = One Button Dialog(message="ERROR!\nData is empty or exist") -> ()  [unwired: 1 in, 1 out]
              }
            }
          }
        }
      }
      event "NO.": Value Change {
        n178 = event-data() -> ("NewVal"=w912:string)  [unwired: 1 in, 5 out]
        n179 = property on="NO." class="CmbBox"() -> ("Strings[]"=w913:string[])  [unwired: 2 in, 2 out]
        n180 = Search 1D Array(1D array=w913, element=w912) -> (index of element=w911:i32)  [unwired: 1 in]
        n181 = case shown="0, Default" w911 {
          tunnel: w915 -> [w922 _]
          tunnel: w914 -> [w921 _]
          frame 0, Default {
            n182 = local read "NO."() -> (w917:string)
            n183 = Format Into String(format string="`%s`.`store_inventory_%s`" ("table"), w922, w917) -> (resulting string=w919:string)  [unwired: 2 in, 1 out]
            n184 = call <vilib>:"DB Tools Select Data.vi"("table"=w919, "connection reference"=w921) -> ("error out"=w916:errorcluster, "data"=w918:variant[][])  [unwired: 4 in, 1 out]
            n185 = case shown="No Error" w916 {
              tunnel: w918 -> [w924 _]
              frame No Error {
                n186 = xnode "Database Variant To Data"("database variant"=w924, "type"=string[][] []) -> ("data"=w925:string[][])  [unwired: 1 in, 1 out]
                n187 = local write "Table"(w925) -> ()
              }
              frame Error {
              }
            }
          }
          frame -1 {
          }
        }
      }
      event "QR_CODE (F2)": Value Change {
        w994 = "\\" ("regular expression")
        n188 = event-data() -> ("NewVal"=w998:string)  [unwired: 1 in, 5 out]
        n189 = local write "QR_CODE (F2)"("") -> ()
        n190 = local read "NO."() -> (w990:string)
        n191 = Format Into String(format string="`%s`.`store_inventory_%s`" ("table"), w989, w990) -> (resulting string=w981:string)  [unwired: 2 in, 1 out]
        n192 = call <vilib>:"DB Tools Select Data.vi"("columns"=string[] ["ITEM_CODE", "STOCK", "ACTUAL", "BALANCE"], "table"=w981, "connection reference"=w988) -> ("data"=w987:variant[][], "connection reference out"=w984:T1)  [unwired: 3 in, 1 out]
        n193 = xnode "Database Variant To Data"("database variant"=w987, "type"=T7 []) -> ("data"=w985:T7)  [unwired: 1 in, 1 out]
        n194 = Match Pattern(string=w998, regular expression=w994) -> (before substring=w970:string, after substring=w997:string)  [unwired: 1 in, 2 out]
        n195 = for {
          tunnel: w985 -> [w1184] mode=indexing
          tunnel: w970 -> [w1182]
          tunnel: [w1181] -> w974
          tunnel: [w1180] -> w993
          i -> [w1181]
          stop <- w1180 stop-if-true
          n196 = Unbundle By Name(w1184) -> ("ITEM_CODE"=w1183:string)
          n197 = Equal?(x=w1183, y=w1182) -> (x = y?=w1180:bool)
        }
        n198 = Match Pattern(string=w997, regular expression=w994) -> (after substring=w996:string)  [unwired: 1 in, 3 out]
        n199 = Match Pattern(string=w996, regular expression=w994) -> (after substring=w995:string)  [unwired: 1 in, 3 out]
        n200 = Match Pattern(string=w995, regular expression=w994) -> (before substring=w977:string)  [unwired: 1 in, 3 out]
        n201 = Fract/Exp String To Number(string=w977) -> (number=w992:dbl)  [unwired: 3 in, 1 out]
        n202 = case shown="True" w993 {
          tunnel: w974 -> [w1185 w1202]
          tunnel: w985 -> [w1200 _]
          tunnel: w992 -> [w1197 _]
          tunnel: w984 -> [w1196 w1203]
          tunnel: w989 -> [_ _]
          tunnel: w981 -> [w1192 _]
          tunnel: [w1188 w1203] -> w982
          tunnel: [w1185 w1201] -> w973
          frame True {
            n203 = Index Array(array=w1200, index=w1185) -> (element=w1199:T11)
            n204 = Unbundle By Name(w1199) -> ("ITEM_CODE"=w1189:string, "STOCK"=w1186:dbl, "ACTUAL"=w1198:dbl)  [unwired: 1 out]
            n205 = Add(x=w1198, y=w1197) -> (x+y=w1187:dbl)
            n206 = Subtract(x=w1187, y=w1186) -> (x-y=w1194:dbl)
            n207 = Format Into String(format string="WHERE ITEM_CODE='%s'" ("table"), w1189) -> (resulting string=w1190:string)  [unwired: 2 in, 1 out]
            n208 = Bundle(w1187, w1194) -> (w1193:cluster{dbl, dbl})  [unwired: 1 in]
            n209 = call <vilib>:"DB Tools Update Data.vi"("condition"=w1190, "data"=w1193, "columns"=string[] ["ACTUAL", "BALANCE"], "table"=w1192, "connection reference"=w1196) -> ("connection reference out"=w1188:T1)  [unwired: 5 in, 1 out]
          }
          frame False {
            n210 = Increment(x=w1202) -> (x+1=w1201:i32)
          }
        }
        n211 = call <vilib>:"DB Tools Select Data.vi"("table"=w981, "connection reference"=w982) -> ("data"=w983:variant[][])  [unwired: 4 in, 2 out]
        n212 = Bundle By Name(cluster=T2 {"Row"=0, "Column"=0} ("Index Values"), "Row"=w973) -> (w975:T2)
        n213 = property on="Table" class="Tbl (strict)"("Index Values"=w975) -> ()  [unwired: 2 in, 2 out]
        n214 = xnode "Database Variant To Data"("database variant"=w983, "type"=string[][] []) -> ("data"=w979:string[][])  [unwired: 1 in, 1 out]
        n215 = flat-sequence {
          tunnel: w979 -> [w1001]
          tunnel: [TRUE ("Key Focus")] -> w971
          frame #0 {
            n216 = local write "Table"(w1001) -> ()
            n217 = Wait (ms)(milliseconds to wait=u32 10) -> ()  [unwired: 1 out]
          }
        }
        n218 = property on="QR_CODE (F2)" class="Str"("Key Focus"=w971) -> ()  [unwired: 2 in, 2 out]
      }
      event Timeout {
        n219 = event-data() -> ()  [unwired: 1 in, 3 out]
        n220 = local read "NO."() -> (w1204:string)
        n221 = Empty String/Path?(string/path=w1204) -> (empty?=w1205:bool)
        n222 = case shown="False" w1205 {
          tunnel: w1204 -> [w1214 _]
          tunnel: w1207 -> [w1210 _]
          tunnel: w1206 -> [w1209 _]
          frame False {
            n223 = Format Into String(format string="`%s`.`STORE_inventory_%s`" ("table"), w1209, w1214) -> (resulting string=w1208:string)  [unwired: 2 in, 1 out]
            n224 = call <vilib>:"DB Tools Select Data.vi"("table"=w1208, "connection reference"=w1210) -> ("data"=w1213:variant[][])  [unwired: 4 in, 2 out]
            n225 = xnode "Database Variant To Data"("database variant"=w1213, "type"=string[][] []) -> ("data"=w1211:string[][])  [unwired: 1 in, 1 out]
            n226 = local write "Table"(w1211) -> ()
          }
          frame True {
          }
        }
      }
    }
  }
